vi "create_z_intensity_tuples.vi"(8 "error in (no error)":errorcluster, 10 "z points":dbl[unit][](array[numeric]), 11 "TrajectoryAK101022Resonance in":refnum<class "TrajectoryAK101022Resonance.lvclass">) -> (0 "error out":errorcluster, 3 "TrajectoryAK101022Resonance out":refnum<class "TrajectoryAK101022Resonance.lvclass">)   [LabVIEW 2010, in "TrajectoryAK101022Resonance.lvclass"]
uses:
  TrajectoryAK101022Resonance.lvclass
  TrajectoryAK101022Resonance.lvclass/TrajectoryAK101022Resonance.ctl
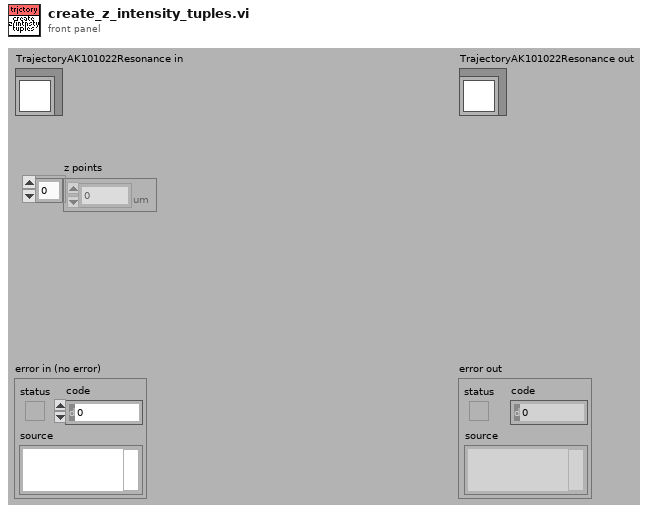
[diagram p1: front panel]
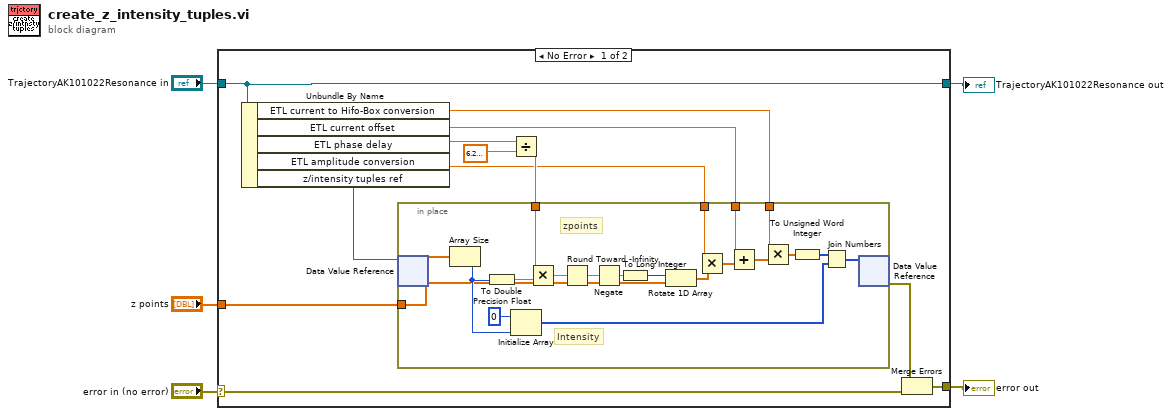
[diagram p0: block diagram]
diagram:
  n1 = case shown="No Error" "error in (no error)" {
    selector: "error in (no error)" -> [w16 w38]
    tunnel: [w15 w38] -> w4
    tunnel: [w14 w37] -> w2
    tunnel: "TrajectoryAK101022Resonance in" -> [w14 w37]
    tunnel: "z points" -> [w9 _]
    frame No Error {
      n2 = Unbundle By Name(w14) -> ("ETL current to Hifo-Box conversion"=w7:dbl[unit], "ETL current offset"=w6:dbl[unit], "ETL phase delay"=w13:dbl[unit], "ETL amplitude conversion"=w10:dbl[unit], "z/intensity tuples ref"=w8:refnum<data-value>)
      n3 = Divide(x=w13, y=dbl[unit] 6.283185307179586) -> (x/y=w11:dbl)
      n4 = in-place {
        in-place-border: w11 -> [w33]
        in-place-border: w10 -> [w29]
        in-place-border: w7 -> [w28]
        in-place-border: w9 -> [w23]
        in-place-border: w6 -> [w19]
        # "Intensity"
        # "zpoints"
        n5 = in-place-dvr #1(w8) -> ()  [unwired: 2 out]
        n6 = Array Size(array=w23) -> (size(s)=w30:i32)
        n7 = To Double Precision Float(number=w30) -> (double precision float=w31:dbl)
        n8 = Initialize Array(u16 0 ("index"), w30) -> (w34:u16[])
        n9 = Multiply(x=w33, y=w31) -> (x*y=w32:dbl)
        n10 = Round Toward -Infinity(1:w32) -> (0:w22:dbl)
        n11 = Negate(x=w22) -> (-x=w21:dbl)
        n12 = To Long Integer(number=w21) -> (32bit integer=w24:i32)
        n13 = Rotate 1D Array(1:w23, 2:w24) -> (0:w25:dbl[unit][])
        n14 = Multiply(x=w29, y=w25) -> (x*y=w20:dbl[unit][])
        n15 = Add(x=w19, y=w20) -> (x+y=w18:dbl[unit][])
        n16 = Multiply(x=w28, y=w18) -> (x*y=w27:dbl[])
        n17 = To Unsigned Word Integer(number=w27) -> (unsigned 16bit integer=w26:u16[])
        n18 = Join Numbers(hi=w26, lo=w34) -> ((hi.lo)=w35:u32[])
        n19 = in-place-dvr #1(w35) -> (w17:errorcluster)  [unwired: 1 out]
      }
      n20 = Merge Errors(w17, w16) -> (w15:errorcluster)
    }
    frame Error {
    }
  }
  "error out" <- w4
  "TrajectoryAK101022Resonance out" <- w2
